vi "07-初级计算器.vi"() -> ()   [LabVIEW 2025]
panel:
  in  "除":bool
  in  "乘":bool
  in  "减":bool
  in  "加":bool
  out "结果":dbl
  in  "输入2":dbl
  in  "输入1":dbl
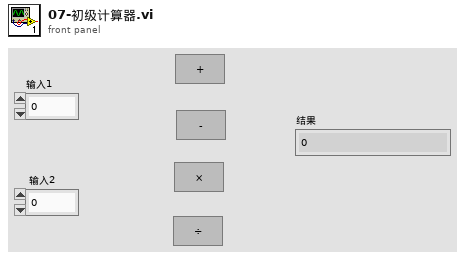
[diagram p1: front panel]
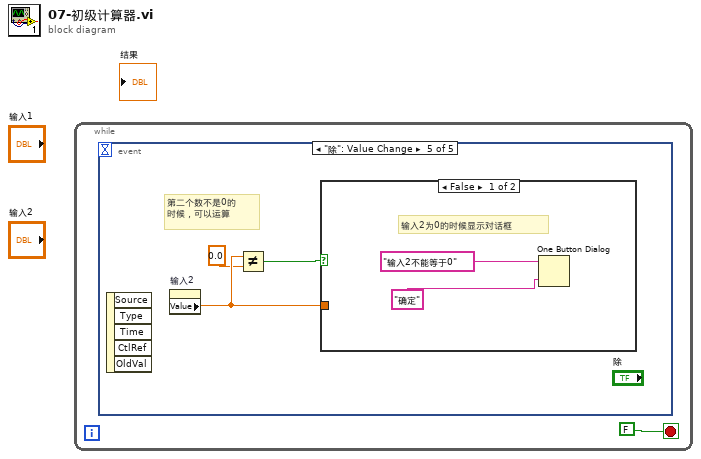
[diagram p0: block diagram]
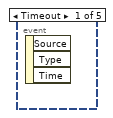
[diagram p2: hidden frame]
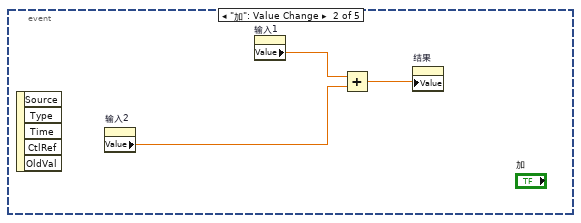
[diagram p3: hidden frame]
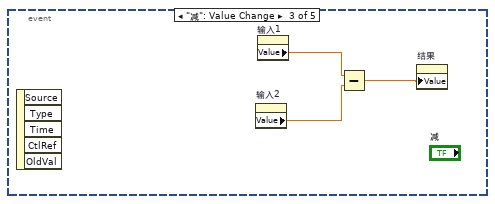
[diagram p4: hidden frame]
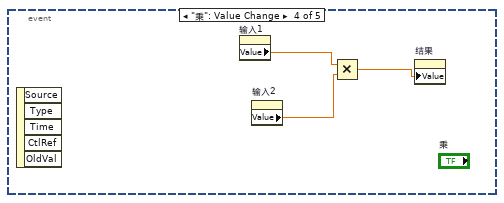
[diagram p5: hidden frame]
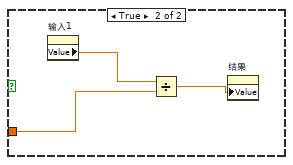
[diagram p6: hidden frame]
diagram:
  n1 = while {
    stop <- FALSE stop-if-true
    n2 = event shown="[4] \"除\": Value Change" {
      selector: _ -> [_ _ _ _ _]
      dyn-events: _ -> [_ _ _ _ _]
      timeout: _ -> [_ _ _ _ _]
      event Timeout {
        n3 = event-data() -> ()  [unwired: 1 in, 3 out]
      }
      event "加": Value Change {
        n4 = event-data() -> ()  [unwired: 1 in, 5 out]
        n5 = property on="输入2" class="DigNum (strict)"() -> ("Value"=w3:dbl)  [unwired: 2 in, 2 out]
        n6 = property on="输入1" class="DigNum (strict)"() -> ("Value"=w4:dbl)  [unwired: 2 in, 2 out]
        n7 = Add(x=w4, y=w3) -> (x+y=w2:dbl)
        n8 = property on="结果" class="DigNum (strict)"("Value"=w2) -> ()  [unwired: 2 in, 2 out]
      }
      event "减": Value Change {
        n9 = event-data() -> ()  [unwired: 1 in, 5 out]
        n10 = property on="输入2" class="DigNum (strict)"() -> ("Value"=w6:dbl)  [unwired: 2 in, 2 out]
        n11 = property on="输入1" class="DigNum (strict)"() -> ("Value"=w7:dbl)  [unwired: 2 in, 2 out]
        n12 = Subtract(x=w7, y=w6) -> (x-y=w5:dbl)
        n13 = property on="结果" class="DigNum (strict)"("Value"=w5) -> ()  [unwired: 2 in, 2 out]
      }
      event "乘": Value Change {
        n14 = event-data() -> ()  [unwired: 1 in, 5 out]
        n15 = property on="输入1" class="DigNum (strict)"() -> ("Value"=w10:dbl)  [unwired: 2 in, 2 out]
        n16 = property on="输入2" class="DigNum (strict)"() -> ("Value"=w9:dbl)  [unwired: 2 in, 2 out]
        n17 = Multiply(x=w10, y=w9) -> (x*y=w8:dbl)
        n18 = property on="结果" class="DigNum (strict)"("Value"=w8) -> ()  [unwired: 2 in, 2 out]
      }
      event "除": Value Change {
        # "第二个数不是0的\n时候，可以运算"
        n19 = event-data() -> ()  [unwired: 1 in, 5 out]
        n20 = property on="输入2" class="DigNum (strict)"() -> ("Value"=w13:dbl)  [unwired: 2 in, 2 out]
        n21 = Not Equal?(x=w13, y=0.0 ("x")) -> (x != y?=w11:bool)
        n22 = case shown="False" w11 {
          tunnel: w13 -> [_ w18]
          frame False {
            # "输入2为0的时候显示对话框"
            n23 = One Button Dialog(message="输入2不能等于0", button name ("OK")="确定" ("message")) -> ()  [unwired: 1 out]
          }
          frame True {
            n24 = property on="输入1" class="DigNum (strict)"() -> ("Value"=w16:dbl)  [unwired: 2 in, 2 out]
            n25 = Divide(x=w16, y=w18) -> (x/y=w17:dbl)
            n26 = property on="结果" class="DigNum (strict)"("Value"=w17) -> ()  [unwired: 2 in, 2 out]
          }
        }
      }
    }
  }
